vi "wiring_array_to_tdms_properties.vi"(11 "wiring":string[][](array[string])=[["    Electrode 1", " Lockin 1", " ", " KH 1: Ground", " 10x", " Open"], ["    Electrode 2", " Lockin 2", " ", " KH 2: Ground", " 10x", " Open"], ["    Electrode 3", " Lockin 3", " I+", " KH 3: Differential", " 10x", " 50k Ohms"], ["    Electrode 4", " Lockin 4", " I-", " KH 4: Differential", " 10x", " 50k Ohms"], ["    Electrode 5", " Lockin 5", " V1-", " KH 5: SE+ (-gnd)", " 10x", " Open"], ["    Electrode 27", " Lockin 7", " Vbg", " KH 7: Differential", " 10x", " 50k Ohms"], ["    Electrode 28", " Lockin 8", " V1+", " KH 8: SE+ (-gnd)", " 10x", " Open"]]) -> (2 "property values":variant[](array[variant]), 3 "property names":string[](array[string]))   [LabVIEW 2016]
uses:
  <vilib>/JDP Science/JDP Science Common Utilities/JDP Utility.lvlib
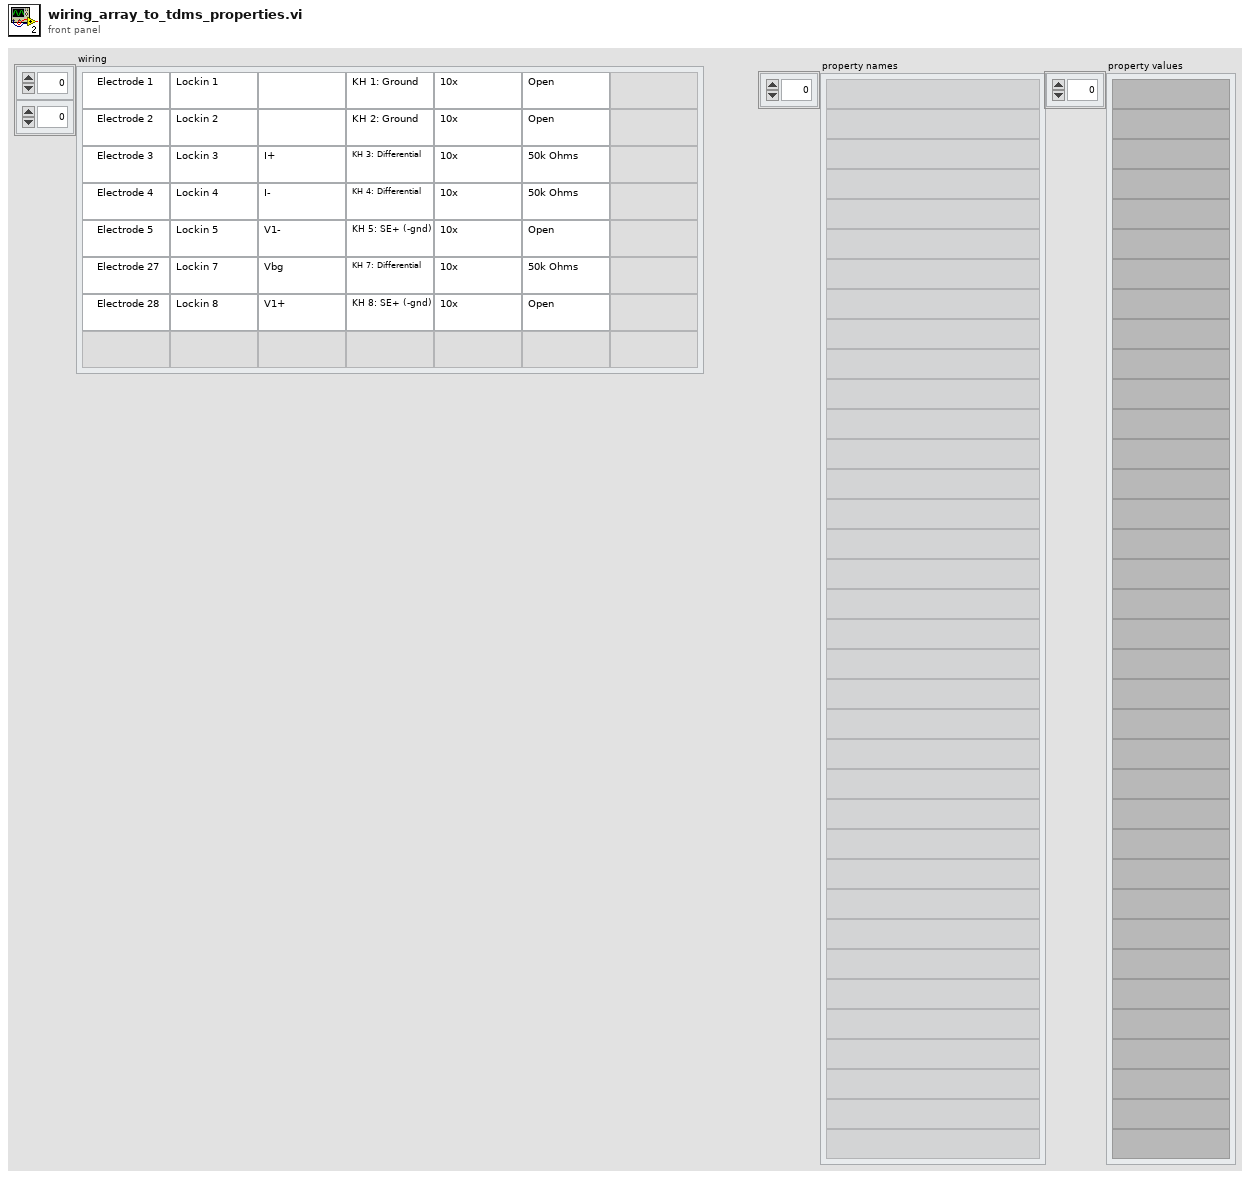
[diagram p1: front panel]
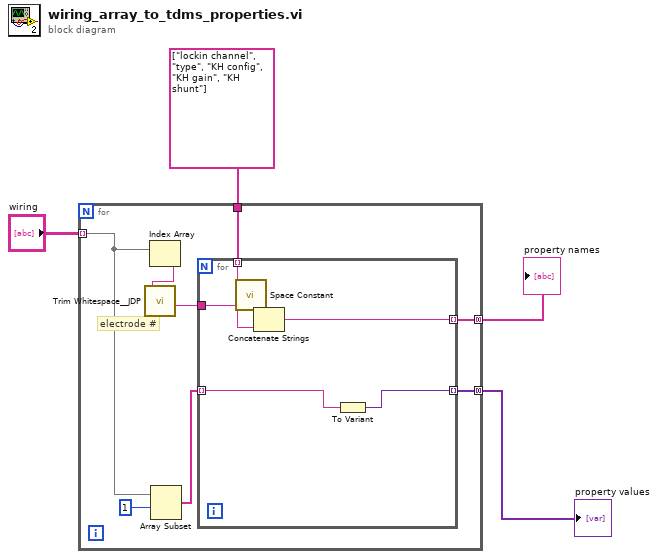
[diagram p0: block diagram]
diagram:
  n1 = for {
    tunnel: "wiring" -> [w11] mode=indexing
    tunnel: string[] ["lockin channel", "type", "KH config", "KH gain", "KH shunt"] -> [w7]
    tunnel: [w6] -> w2 mode=concatenating
    tunnel: [w5] -> w1 mode=concatenating
    # "electrode #"
    n2 = Index Array(array=w11) -> (element=w10:string)  [unwired: 1 in]
    n3 = call <vilib>:"Trim Whitespace__JDP.vi"("String in"=w10) -> ("String out"=w9:string)  [unwired: 6 in]
    n4 = Array Subset(array=w11, index=1) -> (w8:string[])  [unwired: 1 in]
    n5 = for {
      tunnel: w9 -> [w18]
      tunnel: w8 -> [w14] mode=indexing
      tunnel: w7 -> [w17] mode=indexing
      tunnel: [w15] -> w6 mode=indexing
      tunnel: [w13] -> w5 mode=indexing
      n6 = call <vilib>:"Space Constant.vi"() -> ("String"=w16:string)
      n7 = Concatenate Strings(w18, w16, w17) -> (w15:string)
      n8 = To Variant(anything=w14) -> (Variant=w13:variant)
    }
  }
  "property names" <- w2
  "property values" <- w1
